vi "Program08.vi"() -> ()   [LabVIEW 2020]
panel:
  out "String":string
  in  "Ring":u16(ring) items=["A", "B", "C", "D"]
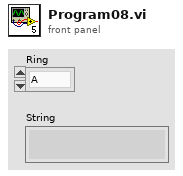
[diagram p1: front panel]
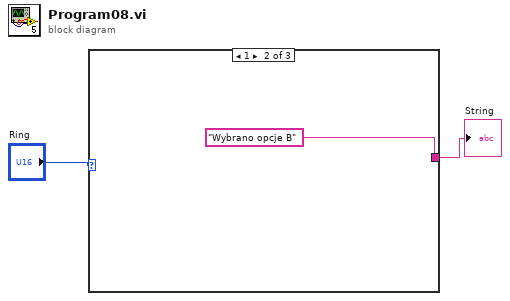
[diagram p0: block diagram]
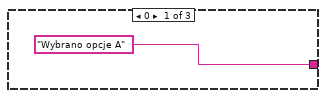
[diagram p2: hidden frame]
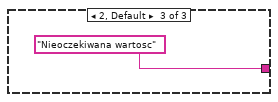
[diagram p3: hidden frame]
diagram:
  n1 = case shown="1" "Ring" {
    tunnel: ["Wybrano opcje A" "Wybrano opcje B" "Nieoczekiwana wartosc"] -> w1
    frame 0 {
    }
    frame 1 {
    }
    frame 2, Default {
    }
  }
  "String" <- w1
